vi "Launch cRIO Vacuum Actor.vi"(5 "DedicatedEnQrs":refnum<queue>, 7 "Vacuum StateQ":refnum<queue>, 8 "error in (no error)":errorcluster, 10 "Caller Actor in":refnum<class "Actor.lvclass">, 11 "cRIO Vacuum in":refnum<class "cRIO Vacuum.lvclass">) -> (0 "error out":errorcluster, 3 "Caller-To-Actor Enqueuer":refnum<class "Message Enqueuer.lvclass">)   [LabVIEW 2015, in "cRIO-Carbondioxide.lvlib" / "CO2-Actor.lvlib" / "cRIO Vacuum.lvclass"]
uses:
  cRIO Vacuum.lvclass
  <vilib>/ActorFramework/Message Enqueuer/Message Enqueuer.lvclass
  <vilib>/ActorFramework/Actor/Actor.lvclass
  Controls/Dedicated Enqueuers.ctl
  Controls/Vacuum State Cluster.ctl
  Controls/Vacuum State Enumerator.ctl
  CO2 Actor/CO2 Actor.lvclass
  cRIO Vacuum.lvclass/cRIO Vacuum.ctl
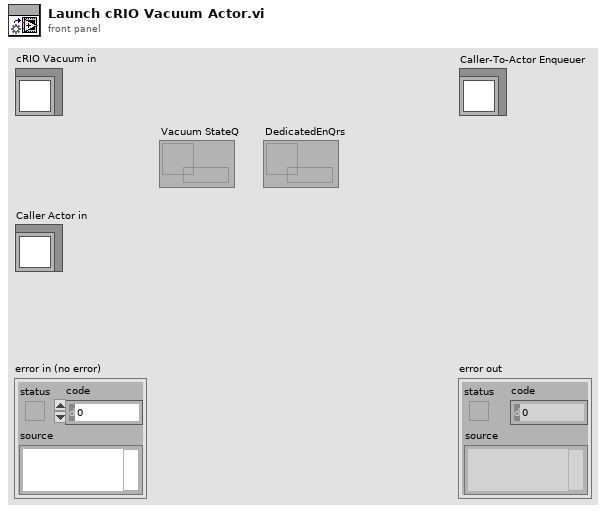
[diagram p1: front panel]
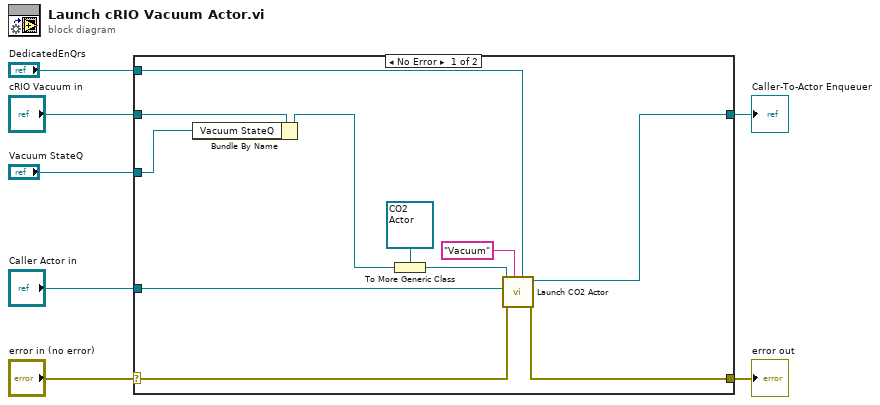
[diagram p0: block diagram]
diagram:
  n1 = case shown="No Error" "error in (no error)" {
    selector: "error in (no error)" -> [w16 w19]
    tunnel: [w15 w19] -> w6
    tunnel: [w10 _] -> w4
    tunnel: "cRIO Vacuum in" -> [w11 _]
    tunnel: "Caller Actor in" -> [w18 _]
    tunnel: "DedicatedEnQrs" -> [w17 _]
    tunnel: "Vacuum StateQ" -> [w8 _]
    frame No Error {
      n2 = Bundle By Name(cluster=w11, "Vacuum StateQ"=w8) -> (w9:refnum<class "cRIO Vacuum.lvclass">)
      n3 = To More Generic Class(target class=refnum<class "CO2 Actor.lvclass"> refnum ("CO2 Actor in"), reference=w9) -> (generic class reference=w13:refnum<class "CO2 Actor.lvclass">)
      n4 = call "Launch CO2 Actor.vi"("DedicatedEnQrs"=w17, "Name"="Vacuum", "error in (no error)"=w16, "Caller Actor in"=w18, "CO2 Actor in"=w13) -> ("error out"=w15:errorcluster, "Caller-To-Actor Enqueuer"=w10:refnum<class "Message Enqueuer.lvclass">)  [unwired: 5 in]
    }
    frame Error {
    }
  }
  "error out" <- w6
  "Caller-To-Actor Enqueuer" <- w4
